vi "LabU.vi"(0 "Serial Com":refnum<visa-resource-name>, 2 "Function":string(combo), 11 "error in (no error)":errorcluster, 12 "Data(PWM)":string) -> (4 "Serial Out":refnum<visa-resource-name>, 8 "result":string, 13 "ok?":bool, 15 "error out":errorcluster)   [LabVIEW 2015]
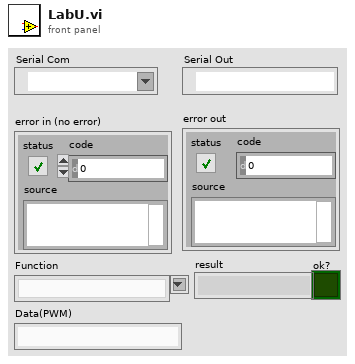
[diagram p1: front panel]
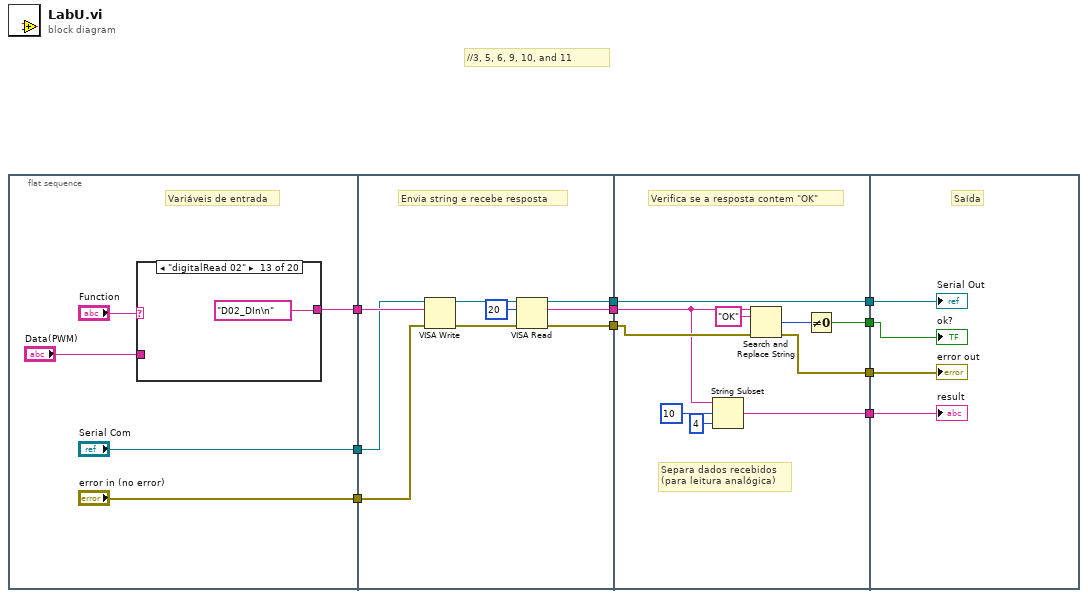
[diagram p0: block diagram]
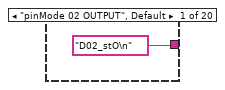
[diagram p2: hidden frame]
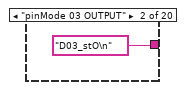
[diagram p3: hidden frame]
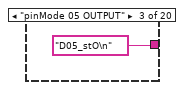
[diagram p4: hidden frame]
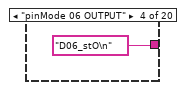
[diagram p5: hidden frame]
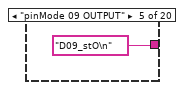
[diagram p6: hidden frame]
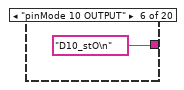
[diagram p7: hidden frame]
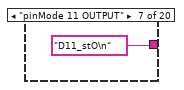
[diagram p8: hidden frame]
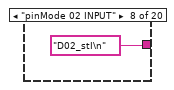
[diagram p9: hidden frame]
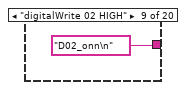
[diagram p10: hidden frame]
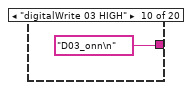
[diagram p11: hidden frame]
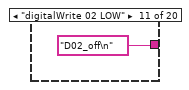
[diagram p12: hidden frame]
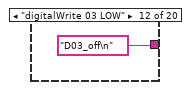
[diagram p13: hidden frame]
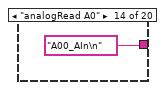
[diagram p14: hidden frame]
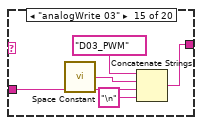
[diagram p15: hidden frame]
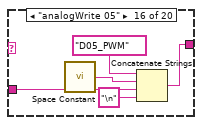
[diagram p16: hidden frame]
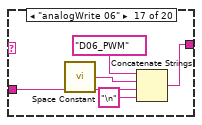
[diagram p17: hidden frame]
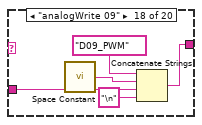
[diagram p18: hidden frame]
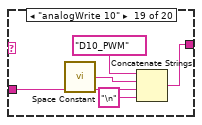
[diagram p19: hidden frame]
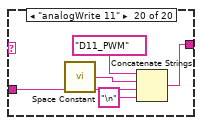
[diagram p20: hidden frame]
diagram:
  # "//3, 5, 6, 9, 10, and 11"
  n1 = flat-sequence {
    tunnel: [w12] -> w10
    tunnel: ["Serial Com"] -> w9
    tunnel: ["error in (no error)"] -> w8
    tunnel: w10 -> [w65]
    tunnel: w9 -> [w64]
    tunnel: w8 -> [w63]
    tunnel: [w62] -> w7
    tunnel: [w61] -> w6
    tunnel: [w60] -> w5
    tunnel: w7 -> [w74]
    tunnel: w6 -> [w73]
    tunnel: w5 -> [w72]
    tunnel: [w72] -> w4
    tunnel: [w71] -> w3
    tunnel: [w70] -> w2
    tunnel: [w69] -> w1
    tunnel: w4 -> [w82]
    tunnel: w3 -> [w81]
    tunnel: w2 -> [w80]
    tunnel: w1 -> [w79]
    frame #0 {
      # "Variáveis de entrada"
      n2 = case shown="\"digitalRead 02\"" "Function" {
        tunnel: ["D02_stO\n" ("write buffer") "D03_stO\n" ("write buffer") "D05_stO\n" ("write buffer") "D06_stO\n" ("write buffer") "D09_stO\n" ("write buffer") "D10_stO\n" ("write buffer") "D11_stO\n" ("write buffer") "D02_stI\n" ("write buffer") "D02_onn\n" ("write buffer") "D03_onn\n" ("write buffer") "D02_off\n" ("write buffer") "D03_off\n" ("write buffer") "D02_DIn\n" ("write buffer") "A00_AIn\n" ("write buffer") w33 w38 w43 w48 w53 w58] -> w12
        tunnel: "Data(PWM)" -> [_ _ _ _ _ _ _ _ _ _ _ _ _ _ w31 w36 w41 w46 w51 w56]
        frame "pinMode 02 OUTPUT", Default {
        }
        frame "pinMode 03 OUTPUT" {
        }
        frame "pinMode 05 OUTPUT" {
        }
        frame "pinMode 06 OUTPUT" {
        }
        frame "pinMode 09 OUTPUT" {
        }
        frame "pinMode 10 OUTPUT" {
        }
        frame "pinMode 11 OUTPUT" {
        }
        frame "pinMode 02 INPUT" {
        }
        frame "digitalWrite 02 HIGH" {
        }
        frame "digitalWrite 03 HIGH" {
        }
        frame "digitalWrite 02 LOW" {
        }
        frame "digitalWrite 03 LOW" {
        }
        frame "digitalRead 02" {
        }
        frame "analogRead A0" {
        }
        frame "analogWrite 03" {
          n3 = call <vilib>:"Space Constant.vi"() -> ("String"=w32:string)
          n4 = Concatenate Strings("D03_PWM" ("write buffer"), w32, w31, "\n" ("string")) -> (w33:string)
        }
        frame "analogWrite 05" {
          n5 = call <vilib>:"Space Constant.vi"() -> ("String"=w37:string)
          n6 = Concatenate Strings("D05_PWM" ("write buffer"), w37, w36, "\n" ("string")) -> (w38:string)
        }
        frame "analogWrite 06" {
          n7 = call <vilib>:"Space Constant.vi"() -> ("String"=w42:string)
          n8 = Concatenate Strings("D06_PWM" ("write buffer"), w42, w41, "\n" ("string")) -> (w43:string)
        }
        frame "analogWrite 09" {
          n9 = call <vilib>:"Space Constant.vi"() -> ("String"=w47:string)
          n10 = Concatenate Strings("D09_PWM" ("write buffer"), w47, w46, "\n" ("string")) -> (w48:string)
        }
        frame "analogWrite 10" {
          n11 = call <vilib>:"Space Constant.vi"() -> ("String"=w52:string)
          n12 = Concatenate Strings("D10_PWM" ("write buffer"), w52, w51, "\n" ("string")) -> (w53:string)
        }
        frame "analogWrite 11" {
          n13 = call <vilib>:"Space Constant.vi"() -> ("String"=w57:string)
          n14 = Concatenate Strings("D11_PWM" ("write buffer"), w57, w56, "\n" ("string")) -> (w58:string)
        }
      }
    }
    frame #1 {
      # "Envia string e recebe resposta"
      n15 = VISA Write(VISA resource name=w64, write buffer=w65, error in (no error)=w63) -> (VISA resource name out=w67:refnum<visa-resource-name>, error out=w66:errorcluster)  [unwired: 1 out]
      n16 = VISA Read(VISA resource name=w67, byte count=u32 20, error in (no error)=w66) -> (VISA resource name out=w60:refnum<visa-resource-name>, read buffer=w61:string, error out=w62:errorcluster)  [unwired: 1 out]
    }
    frame #2 {
      # "Separa dados recebidos\n(para leitura analógica)"
      # "Verifica se a resposta contem \"OK\""
      n17 = String Subset(string=w73, offset (0)=10, length (rest)=4 ("length (rest)")) -> (substring=w69:string)
      n18 = Search and Replace String(input string=w73, search string="OK", error in=w74) -> (number of replacements=w75:i32, error out=w70:errorcluster)  [unwired: 5 in, 2 out]
      n19 = Not Equal To 0?(x=w75) -> (x != 0?=w71:bool)
    }
    frame #3 {
      # "Saída"
      "error out" <- w80
      "ok?" <- w81
      "result" <- w79
      "Serial Out" <- w82
    }
  }
